vi "setDescription.vi"(8 "error in (no error)":errorcluster, 10 "description":string="Unknown", 11 "Espresso in":refnum<class "Espresso.lvclass">) -> (0 "error out":errorcluster, 3 "Espresso out":refnum<class "Espresso.lvclass">)   [LabVIEW 2016, in "Espresso.lvclass"]
uses:
  Espresso.lvclass
  Beverage Class/Beverage.lvclass
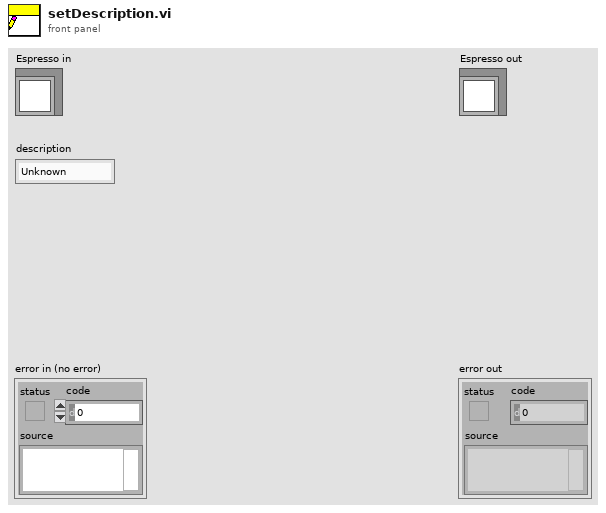
[diagram p1: front panel]
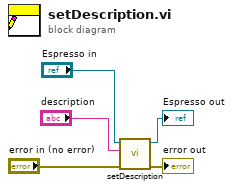
[diagram p0: block diagram]
diagram:
  n1 = call-parent "setDescription.vi"("error in (no error)"="error in (no error)", "description"="description", "Beverage in"="Espresso in") -> ("error out"=→"error out":errorcluster, "Beverage out"=→"Espresso out":refnum<class "Espresso.lvclass">)  [unwired: 7 in]
